vi "dashboard_data_store.vi"(4 "mode":T1(ring), 7 "joe_johnson_data":T4={"analog"=0.0, "input"=0.0, "joe_johnson_state"=enum."fold", "idg_state"=enum."fault_high"}, 8 "roller data":T7, 9 "drivetrain_data":T8, 10 "gun_slow":T11={"turret"={"turret_analog"=0.0, "turret_angle"=0.0, "turret_motor"=0.0, "turret_idg_state"=enum."fault_high"}, "hood"={"hood_analog"=0.0, "hood_angle"=0.0, "hood_motor"=0.0, "hood_idg_state"=enum."fault_high"}}, 11 "gun_fast":T12) -> ()   [LabVIEW 2011]
uses:
  dashboard_data_gun_fast.ctl
  gun/gun_motor_state.ctl
  gun/gun_tracking_mode.ctl
  gun/gun_rt_slow_upstream_data.ctl
  idg_trust_t.ctl
  dashboard_data_drivetrain.ctl
  drivetrain/gear_shift_state.ctl
  drivetrain/gear_internal_shift_state.ctl
  roller/roller_internal_state.ctl
  roller/roller_user_state.ctl
  joe_johnson/joe_johnson_state.ctl
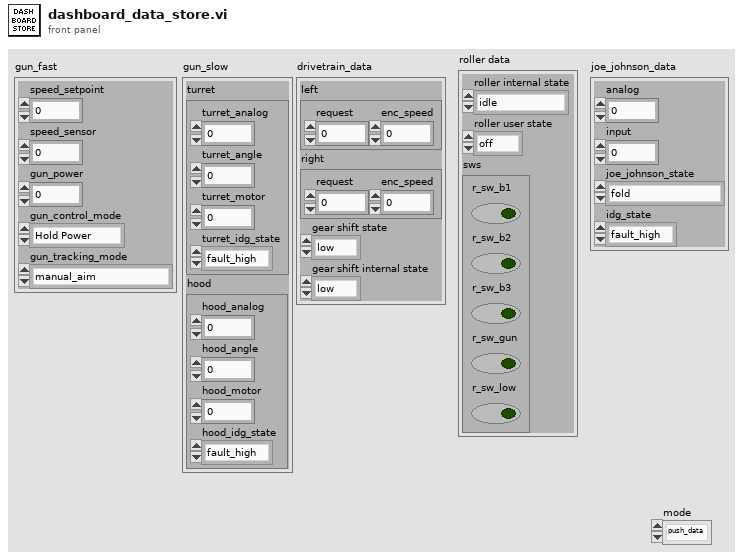
[diagram p1: front panel]
types:
  T1 = enum16{"push_data", "write_joe_johnson", "write_roller", "write_drivetrain", "write_gun_fast", "write_gun_slow"}
  T2 = typedef "joe_johnson_state.ctl" = enum16{"fold", "down", "up", "ramp", "bridge_lift", "manual", "ramp_stay"}
  T3 = typedef "idg_trust_t.ctl" = enum16{"fault_move", "fault_high", "fault_low", "out_high", "out_low", "trust"}
  T4 = cluster{"analog":dbl, "input":dbl, "joe_johnson_state":T2, "idg_state":T3}
  T5 = typedef "roller_internal_state.ctl" = enum16{"idle", "bump", "full", "fire_intermediate", "fire_finish", "fire_entry", "fire_end", "fire_recover"}
  T6 = typedef "roller_user_state.ctl" = enum16{"off", "collect", "blow", "force suck"}
  T7 = cluster{"roller internal state":T5, "roller user state":T6, "sws":cluster{"r_sw_b1":bool, "r_sw_b2":bool, "r_sw_b3":bool, "r_sw_gun":bool, "r_sw_low":bool}}
  T8 = typedef "dashboard_data_drivetrain.ctl" = cluster{"left":cluster{"request":dbl, "enc_speed":dbl}, "right":cluster{"request":dbl, "enc_speed":dbl}, "gear shift state":T9, "gear shift internal state":T10}
  T9 = typedef "gear_shift_state.ctl" = enum16{"low", "high"}
  T10 = typedef "gear_internal_shift_state.ctl" = enum16{"low", "high", "low_peak", "high_peak"}
  T11 = typedef "gun_rt_slow_upstream_data.ctl" = cluster{"turret":cluster{"turret_analog":dbl, "turret_angle":dbl, "turret_motor":dbl, "turret_idg_state":T3}, "hood":cluster{"hood_analog":dbl, "hood_angle":dbl, "hood_motor":dbl, "hood_idg_state":T3}}
  T12 = typedef "dashboard_data_gun_fast.ctl" = cluster{"speed_setpoint":dbl, "speed_sensor":dbl, "gun_power":dbl, "gun_control_mode":T13, "gun_tracking_mode":T14}
  T13 = typedef "gun_motor_state.ctl" = enum16{"Hold Power", "Hold Speed", "Hold Distance", "Stop"}
  T14 = typedef "gun_tracking_mode.ctl" = enum16{"manual_aim", "auto_aim_camera", "preset_center_field", "preset_right_pocket", "preset_left_pocket", "align_center", "align_center_backwards", "auto_aim_key", "align_fold", "auton_custom", "preset_pass", "auto_aim_auton"}
  T15 = cluster{"gun_fast":T12, "gun_slow":T11, "drivetrain_data":T8, "roller data":cluster{"roller internal state":T5, "roller user state":T6, "sws":cluster{"r_sw_b1":bool, "r_sw_b2":bool, "r_sw_b3":bool, "r_sw_gun":bool, "r_sw_low":bool}}, "joe_johnson_data":cluster{"analog":dbl, "input":dbl, "joe_johnson_state":T2, "idg_state":T3}}
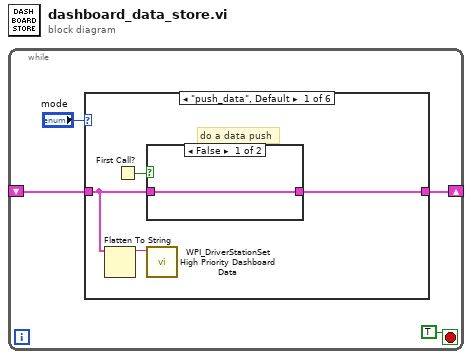
[diagram p0: block diagram]
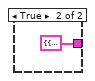
[diagram p2: hidden frame]
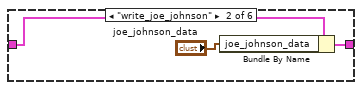
[diagram p3: hidden frame]
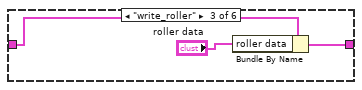
[diagram p4: hidden frame]
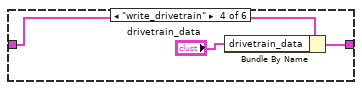
[diagram p5: hidden frame]
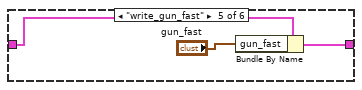
[diagram p6: hidden frame]
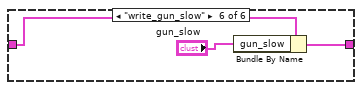
[diagram p7: hidden frame]
diagram:
  n1 = while {
    shift-right: [w3] -> _
    shift-left: _ -> [w2]
    stop <- TRUE stop-if-true
    n2 = case shown="\"push_data\", Default" "mode" {
      tunnel: [w7 w12 w15 w18 w21 w23] -> w3
      tunnel: w2 -> [w5 w13 w16 w19 w22 w24]
      frame "push_data", Default {
        # "do a data push"
        n3 = Flatten To String(anything=w5) -> (data string=w6:string)  [unwired: 3 in, 2 out]
        n4 = First Call?() -> (First Call?: T/F=w8:bool)
        n5 = case shown="False" w8 {
          tunnel: [w9 T15 {"gun_fast"={"speed_setpoint"=0.0, "speed_sensor"=0.0, "gun_power"=0.0, "gun_control_mode"=enum."Hold Power", "gun_tracking_mode"=enum."manual_aim"}, "gun_slow"={"turret"={"turret_analog"=0.0, "turret_angle"=0.0, "turret_motor"=0.0, "turret_idg_state"=enum."fault_high"}, "hood"={"hood_analog"=0.0, "hood_angle"=0.0, "hood_motor"=0.0, "hood_idg_state"=enum."fault_high"}}, "drivetrain_data"={"left"={"request"=0.0, "enc_speed"=0.0}, "right"={"request"=0.0, "enc_speed"=0.0}, "gear shift state"=enum."low", "gear shift internal state"=enum."low"}, "roller data"={"roller internal state"=enum."idle", "roller user state"=enum."off", "sws"={"r_sw_b1"=FALSE, "r_sw_b2"=FALSE, "r_sw_b3"=FALSE, "r_sw_gun"=FALSE, "r_sw_low"=FALSE}}, "joe_johnson_data"={"analog"=0.0, "input"=0.0, "joe_johnson_state"=enum."fold", "idg_state"=enum."fault_high"}} ("dashboard_data")] -> w7
          tunnel: w5 -> [w9 _]
          frame False {
          }
          frame True {
          }
        }
        n6 = call <vilib>:"WPI_DriverStationSet High Priority Dashboard Data.vi"("User Data"=w6) -> ()  [unwired: 10 in, 1 out]
      }
      frame "write_joe_johnson" {
        n7 = Bundle By Name(cluster=w13, "joe_johnson_data"="joe_johnson_data") -> (w12:T15)
      }
      frame "write_roller" {
        n8 = Bundle By Name(cluster=w16, "roller data"="roller data") -> (w15:T15)
      }
      frame "write_drivetrain" {
        n9 = Bundle By Name(cluster=w19, "drivetrain_data"="drivetrain_data") -> (w18:T15)
      }
      frame "write_gun_fast" {
        n10 = Bundle By Name(cluster=w22, "gun_fast"="gun_fast") -> (w21:T15)
      }
      frame "write_gun_slow" {
        n11 = Bundle By Name(cluster=w24, "gun_slow"="gun_slow") -> (w23:T15)
      }
    }
  }
